vi "AssertRowValue.vi"(0 "VI Reference In":refnum<vi>, 1 "Test Label":string, 2 "delimiter (>>)":string=">>", 3 "Assert Only? (F)":bool, 5 "Control Path":string, 7 "Row Index":i32, 9 "Item Value":string[](array[string]), 11 "Error In":errorcluster, 12 "Assert Interval(10 ms)":u32=10, 13 "Timeout(5 sec)":dbl=5.0) -> (4 "VI Reference Out":refnum<vi>, 6 "Asserted Value":string[](array[string]), 15 "Error Out":errorcluster)   [LabVIEW 2016, in "Drona.lvlib" / "AssertControlValue.lvlib" / "AssertTable.lvlib"]
doc: "Asserts if the values in the specified row of the table control is equal.\n\nThe input control name is given as a string , incase of path, use delimiters inbetween the path.\nThis VI gets the value of the control, untill the value is equal to the input value."
uses:
  AssertTable.lvlib
  Get/GetControlRef/GetControlRefByPath.vi
  <vilib>/Utility/error.llb/Error Cluster From Error Code.vi
  <vilib>/addons/_JKI Toolkits/Caraya/classes/Assert/Assert Equal Value_Variant.vi
  <vilib>/ErrorRing/Error Ring.xnode
  Get/GetControlRef/GetControlRef.lvlib
  <vilib>/addons/_JKI Toolkits/Caraya/classes/Assert/Assert.lvclass
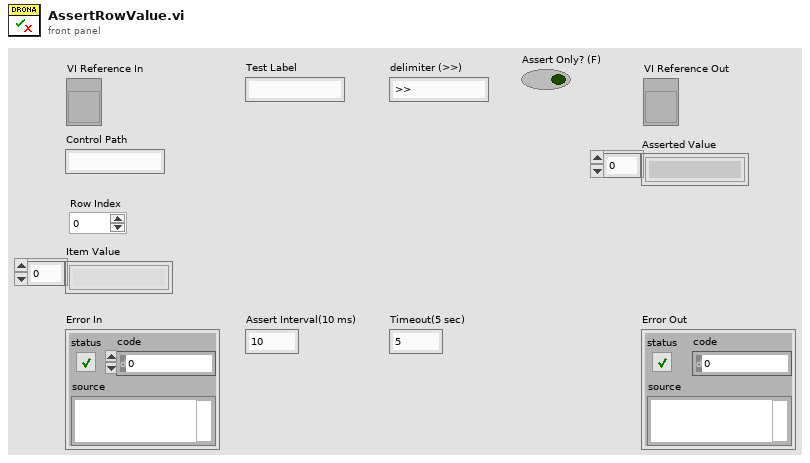
[diagram p1: front panel]
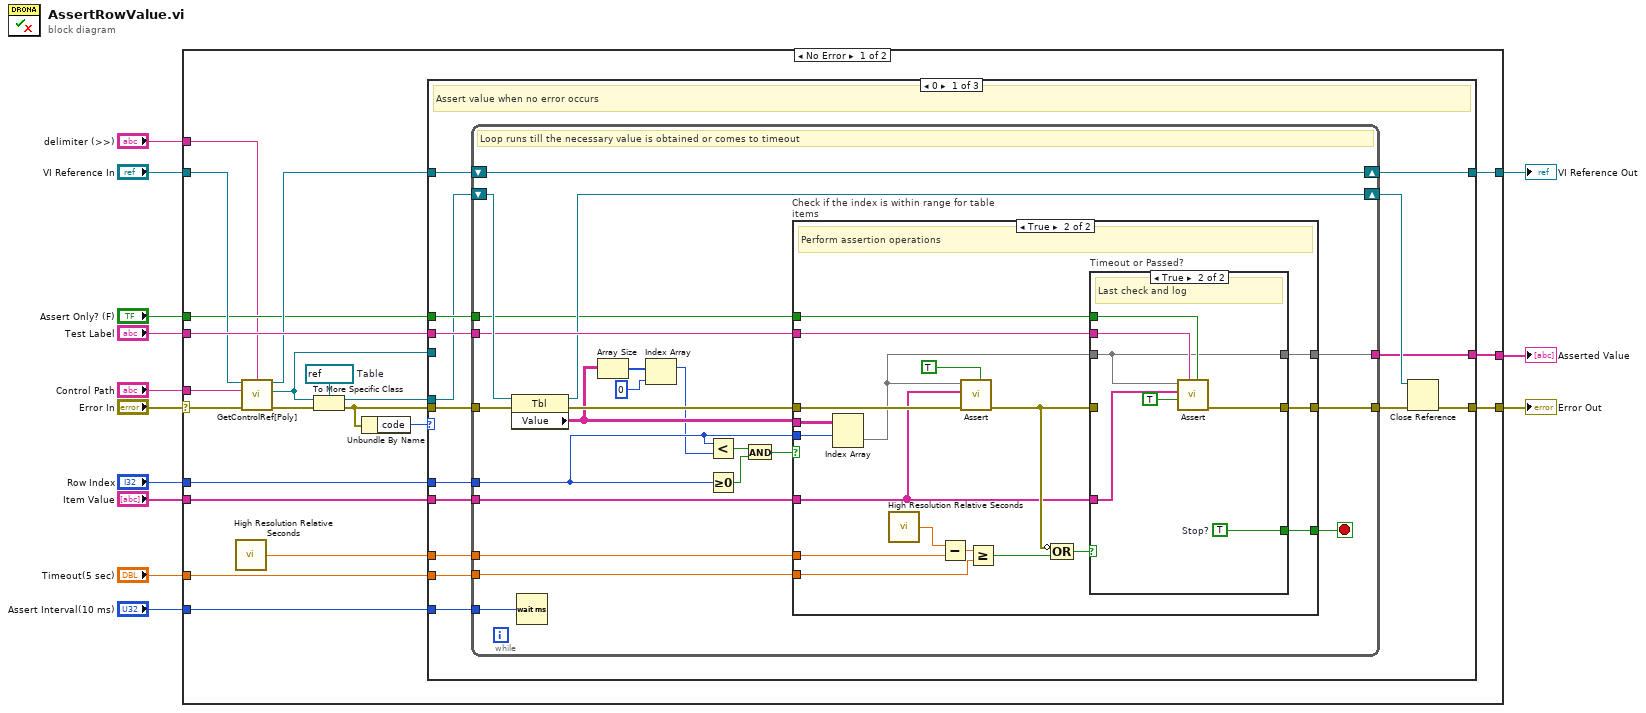
[diagram p0: block diagram]
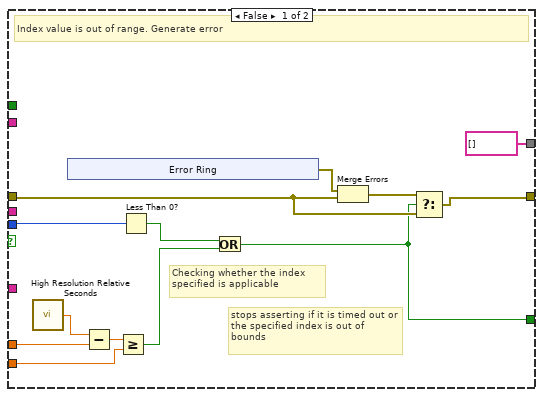
[diagram p2: hidden frame]
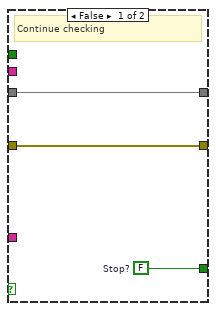
[diagram p3: hidden frame]
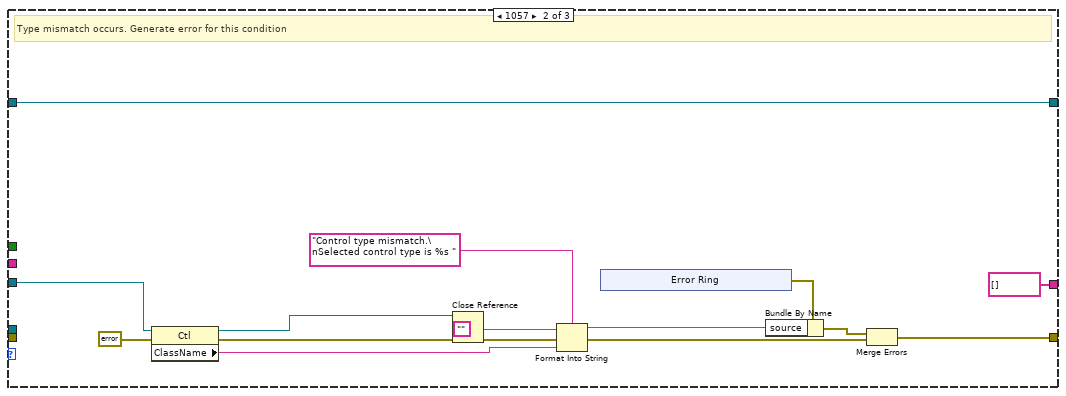
[diagram p4: hidden frame]
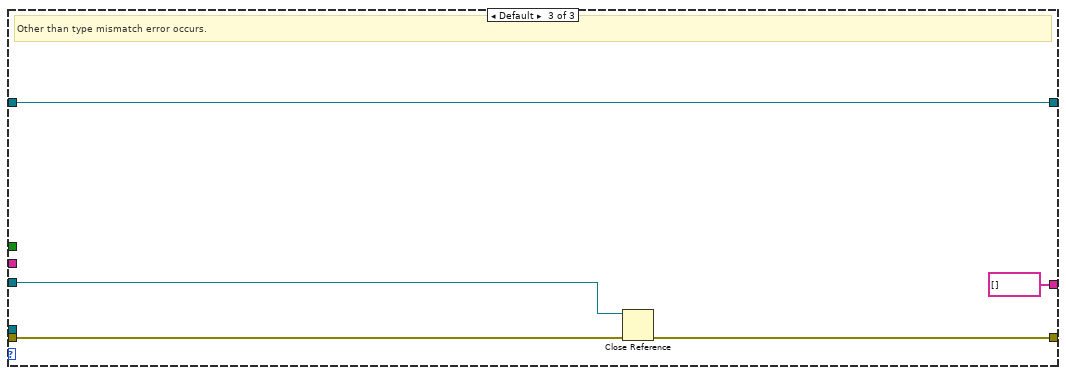
[diagram p5: hidden frame]
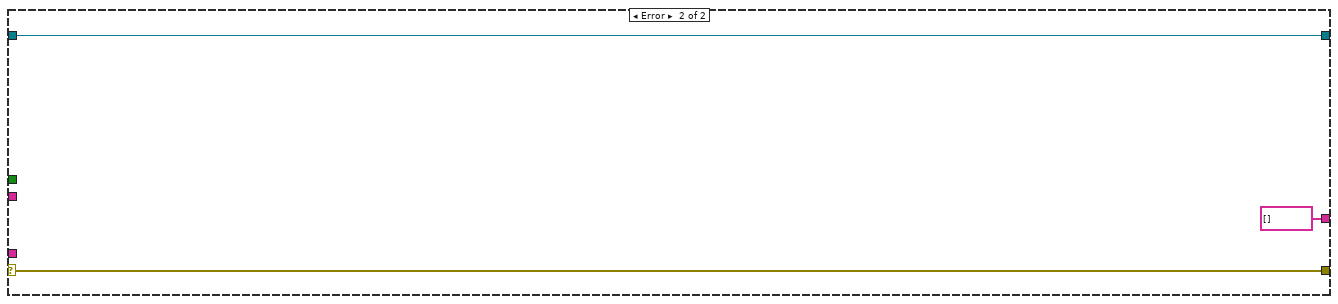
[diagram p6: hidden frame]
diagram:
  n1 = case shown="No Error" "Error In" {
    selector: "Error In" -> [w29 w145]
    tunnel: "Timeout(5 sec)" -> [w34 _]
    tunnel: [w33 w144] -> w12
    tunnel: "Row Index" -> [w32 _]
    tunnel: [w24 w145] -> w11
    tunnel: "Assert Interval(10 ms)" -> [w31 _]
    tunnel: "Test Label" -> [w30 _]
    tunnel: "VI Reference In" -> [w28 w144]
    tunnel: "Control Path" -> [w14 _]
    tunnel: "delimiter (>>)" -> [w15 _]
    tunnel: "Assert Only? (F)" -> [w23 _]
    tunnel: [w22 string[] [] ("Value")] -> w1
    tunnel: "Item Value" -> [w19 _]
    frame No Error {
      w21 = refnum<vi> refnum  # Table
      n2 = call <vilib>:"High Resolution Relative Seconds.vi"() -> ("relative seconds"=w27:dbl)
      n3 = call-poly "GetControlRef[Poly].vi"("VI Reference In"=w28, "delimiter (>>)"=w15, "Control Path"=w14, "error In"=w29) -> ("VI Reference Out"=w25:refnum<vi>, "Ctl Refnum"=w16:refnum<vi>, "error out"=w26:errorcluster)  [unwired: 9 in]
      n4 = To More Specific Class(target class=w21, reference=w16, error in=w26) -> (specific class reference=w20:refnum<vi>, error out=w18:errorcluster)
      n5 = Unbundle By Name(w18) -> ("code"=w17:i32)
      n6 = case shown="0" w17 {
        tunnel: w34 -> [w49 _ _]
        tunnel: [w48 w132 w142] -> w33
        tunnel: w32 -> [w47 _ _]
        tunnel: w31 -> [w45 _ _]
        tunnel: w30 -> [w44 _ _]
        tunnel: w27 -> [w43 _ _]
        tunnel: w25 -> [w42 w132 w142]
        tunnel: [w41 w120 w140] -> w24
        tunnel: w23 -> [w39 _ _]
        tunnel: [w38 string[] [] ("Value") string[] [] ("Value")] -> w22
        tunnel: w18 -> [w37 _ w141]
        tunnel: w20 -> [w36 _ _]
        tunnel: w19 -> [w35 _ _]
        tunnel: w16 -> [_ w119 w139]
        frame 0 {
          # "Assert value when no error occurs"
          n7 = while {
            tunnel: w47 -> [w55]
            tunnel: w49 -> [w70]
            tunnel: w43 -> [w71]
            tunnel: w37 -> [w65]
            tunnel: [w68] -> w46
            tunnel: w45 -> [w66]
            tunnel: w44 -> [w62]
            shift-right: [w63] -> w48
            shift-left: w42 -> [w63]
            shift-right: [w61] -> w40
            shift-left: w36 -> [w64]
            tunnel: w39 -> [w60]
            tunnel: [w59] -> w38
            tunnel: w35 -> [w58]
            stop <- w69 stop-if-true
            # "Loop runs till the necessary value is obtained or comes to timeout"
            n8 = property on="Property Node" class="Tbl"(reference=w64, error in=w65) -> (reference out=w61:refnum<vi>, error out=w67:errorcluster, "Value"=w57:string[][])
            n9 = Wait (ms)(milliseconds to wait=w66) -> ()  [unwired: 1 out]
            n10 = Array Size(array=w57) -> (size(s)=w56:i32[])
            n11 = Index Array(array=w56, index=0) -> (element=w51:i32)
            n12 = Less?(x=w55, y=w51) -> (x < y?=w53:bool)
            n13 = Greater Or Equal To 0?(x=w55) -> (x >= 0?=w54:bool)
            n14 = And(x=w53, y=w54) -> (x .and. y?=w52:bool)
            n15 = case "Check if the index is within range for table items" shown="True" w52 {
              tunnel: w71 -> [w77 w107]
              tunnel: w70 -> [w76 w104]
              tunnel: [w72 w96] -> w69
              tunnel: [w73 w97] -> w68
              tunnel: w62 -> [_ w102]
              tunnel: w60 -> [_ w95]
              tunnel: [string[] [] ("Value") w94] -> w59
              tunnel: w58 -> [_ w93]
              tunnel: w57 -> [_ w92]
              tunnel: w55 -> [w75 w90]
              tunnel: w67 -> [w74 w103]
              frame False {
                # "stops asserting if it is timed out or the specified index is out of bounds"
                # "Checking whether the index specified is applicable"
                # "Index value is out of range. Generate error"
                n16 = call <vilib>:"High Resolution Relative Seconds.vi"() -> ("relative seconds"=w81:dbl)
                n17 = xnode "Error Ring"() -> ("error out"=w83:errorcluster)
                n18 = Subtract(x=w81, y=w77) -> (x-y=w82:dbl)
                n19 = Greater Or Equal?(x=w82, y=w76) -> (x >= y?=w79:bool)
                n20 = Less Than 0?(x=w75) -> (x < 0?=w80:bool)
                n21 = Or(x=w80, y=w79) -> (x .or. y?=w72:bool)
                n22 = Merge Errors(w83, w74) -> (w78:errorcluster)
                n23 = Select(t=w78, s=w72, f=w74) -> (s? t:f=w73:errorcluster)
              }
              frame True {
                # "Perform assertion operations"
                n24 = Index Array(array=w92, index (row)=w90) -> (element=w91:string[])  [unwired: 1 in]
                n25 = call <vilib>:"High Resolution Relative Seconds.vi"() -> ("relative seconds"=w106:dbl)
                n26 = Subtract(x=w106, y=w107) -> (x-y=w105:dbl)
                n27 = call-poly <vilib>:"Assert.vi"("Assert Only? (F)"=TRUE, "error in (no error)"=w103, "Y"=w93, "X"=w91) -> ("error out"=w100:errorcluster)  [unwired: 6 in, 1 out]
                n28 = Greater Or Equal?(x=w105, y=w104) -> (x >= y?=w101:bool)
                n29 = Compound Arithmetic op=OR(invert w100, w101) -> (w99:bool)
                n30 = case "Timeout or Passed?" shown="True" w99 {
                  tunnel: w100 -> [w110 _]
                  tunnel: w93 -> [_ w116]
                  tunnel: w91 -> [w108 w111]
                  tunnel: w102 -> [_ w117]
                  tunnel: [w110 w115] -> w97
                  tunnel: [w109 w114] -> w96
                  tunnel: w95 -> [_ w112]
                  tunnel: [w108 w111] -> w94
                  frame False {
                    w109 = FALSE  # Stop?
                    # "Continue checking"
                  }
                  frame True {
                    w114 = TRUE  # Stop?
                    # "Last check and log"
                    n31 = call-poly <vilib>:"Assert.vi"("Assert Only? (F)"=w112, "Label"=w117, "Register with caller test (F)"=TRUE, "Y"=w116, "X"=w111) -> ("error out"=w115:errorcluster)  [unwired: 5 in, 1 out]
                  }
                }
              }
            }
          }
          n32 = Close Reference(reference=w40, error in (no error)=w46) -> (error out=w41:errorcluster)
        }
        frame 1057 {
          # "Type mismatch occurs. Generate error for this condition"
          n33 = property class="Ctl"(reference=w119, error in=errorcluster {"status"=FALSE, "code"=0, "source"=""} ("error out")) -> (reference out=w121:refnum<vi>, error out=w131:errorcluster, "ClassName"=w128:string)
          n34 = Close Reference(reference=w121, error in (no error)=w131) -> (error out=w122:errorcluster)
          n35 = Format Into String(format string="Control type mismatch.\nSelected control type is %s ", initial string="", error in=w122, w128) -> (resulting string=w125:string, error out=w123:errorcluster)
          n36 = xnode "Error Ring"() -> ("error out"=w126:errorcluster)
          n37 = Bundle By Name(cluster=w126, "source"=w125) -> (w124:errorcluster)
          n38 = Merge Errors(w124, w123) -> (w120:errorcluster)
        }
        frame Default {
          # "Other than type mismatch error occurs."
          n39 = Close Reference(reference=w139, error in (no error)=w141) -> (error out=w140:errorcluster)
        }
      }
    }
    frame Error {
    }
  }
  "Error Out" <- w11
  "VI Reference Out" <- w12
  "Asserted Value" <- w1
